vi "Set Pulse Width and Damping [PDW].vi"(7 "Micropulse # In":i32, 8 "error in (no error)":errorcluster, 9 "Width (ns)":u32, 10 "Damping":T1, 11 "Channel Number":u32) -> (0 "error out":errorcluster, 5 "Micropulse # Out":i32)   [LabVIEW 2026, in "MicroPulse_Driver.lvlib"]
doc: "Selects the damping and pulser width for a given channel (or all channels if <channel> is 0). The settings will apply to all tests using the specified channel as RXN or TXN parameters. There are 8 standard pulse widths (for compatibility with earlier systems) and pulse widths between 16nSec and 1010nSec in 2nSec steps.\n\nParameters:\n<channel> : Integer value from 0 to 24 (0 for all channels).\n\n<damping> : \n0 = 660 ohms\n1 = 458 ohms\n2 = 220 ohms\n3 = 149 ohms\n4 = 102 ohms\n5 = 82 ohms\n6 = 63 ohms\n7 = 51 ohms\n\n<width> :\n0 = 50 nSec\n1 = 100 nSec\n2 = 150 nSec\n3 = 200 nSec\n4 = 250 nSec\n5 = 300 nSec\n6 = 350 nSec\n7 = 225 nSec\n16 – 1010 = Specifies the pulse width in nanoseconds i.e. 30 = 30nSec. Valid every 2nSec step.\n\nDefault: PDW 0 4 3\n\nExample: PDW 1 7 4 : Set pulser/receiver channel 1 to 54ohm damping and 250nSec pulse width.\n\nNote : The damping values given are for MicroPulse 5. The values for LT1, LT2, MPLT and LTPA differ slightly. Contact Peak NDT for more information."
uses:
  MicroPulse_Driver.lvlib
  <instrlib>/MicroPulse/Public/Data/Datatypes/MP - pulse damping.ctl
  Private/MP-Registry Action-Enum.ctl
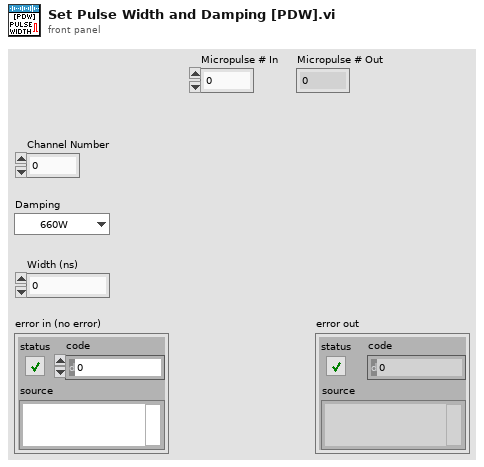
[diagram p1: front panel]
types:
  T1 = typedef "MicroPulse_Driver.lvlib/MP - pulse damping.ctl" = enum16{"660W", "458W", "220W", "149W", "102W", "82W", "63W", "51W"}
  T2 = typedef "MicroPulse_Driver.lvlib/MP-Registry Action-Enum.ctl" = enum16{"Read", "Add Test", "Add Command", "Add Gate Command", "Add Encoder Command", "Clear Command  List", "Set Registry", "Set System Details", "Set DOF", "Set Velocity", "Disable Asynch Reads", "Enable Asynch Reads", "Add Connection", "Disconnect", "Shutdown"}
  T3 = typedef "MicroPulse_Driver.lvlib/TCP config.ctl" = cluster{"Connection ID":refnum<k5>, "IP address":string, "host port":u16, "OC timeout":i32, "Read timeout":i32, "Write timeout":i32}
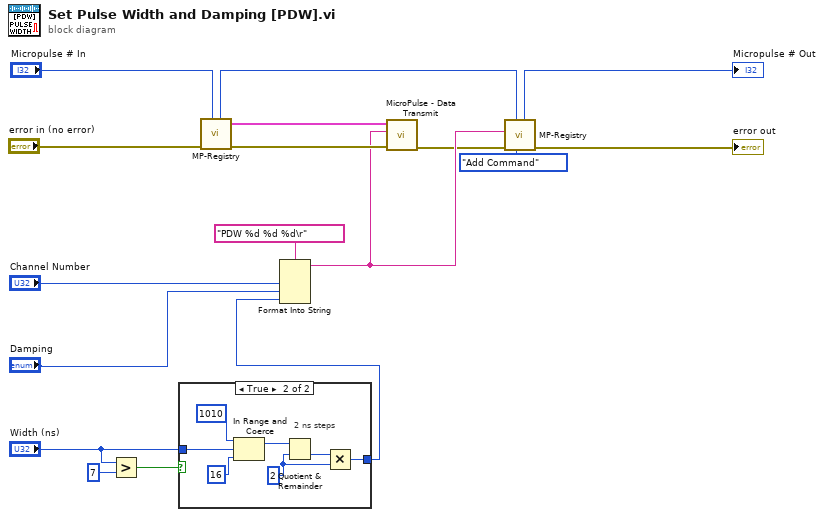
[diagram p0: block diagram]
diagram:
  n1 = Greater?(x="Width (ns)", y=7) -> (0:w3:bool)
  n2 = case shown="True" w3 {
    tunnel: [w18 w20] -> w1
    tunnel: "Width (ns)" -> [w18 w19]
    frame False {
    }
    frame True {
      w21 = 2 ("y")
      # "2 ns steps"
      n3 = In Range and Coerce(upper limit=1010, x=w19, lower limit=16) -> (coerced(x)=w23:u32)  [unwired: 1 out]
      n4 = Quotient & Remainder(x=w23, y=w21) -> (floor(x/y)=w22:u32)  [unwired: 1 out]
      n5 = Multiply(x=w22, y=w21) -> (x*y=w20:u32)
    }
  }
  n6 = call "MP-Registry.vi"("Micropulse # In"="Micropulse # In", "error in (no error)"="error in (no error)") -> ("error out"=w15:errorcluster, "TCP config"=w14:T3, "Micropulse # Out"=w9:i32)  [unwired: 6 in, 1 out]
  n7 = Format Into String(format string="PDW %d %d %d\r", "Channel Number", "Damping", w1) -> (resulting string=w13:string)  [unwired: 2 in, 1 out]
  n8 = call "MicroPulse - Data Transmit.vi"("error in (no error)"=w15, "data"=w13, "TCP config"=w14) -> ("error out"=w11:errorcluster)  [unwired: 6 in, 2 out]
  n9 = call "MP-Registry.vi"("Action"=MP-Registry_Action-Enum."Add Command", "Micropulse # In"=w9, "error in (no error)"=w11, "Data in"=w13) -> ("error out"=→"error out":errorcluster, "Micropulse # Out"=→"Micropulse # Out":i32)  [unwired: 4 in, 2 out]
